vi "Write Page General Properties.vi"(8 "error in (no error)":errorcluster, 10 "General Page Properties":T1, 11 ".NET Refnum in":refnum<k24>) -> (0 "error out":errorcluster, 3 ".NET Refnum out":refnum<k24>)   [LabVIEW 2015, in "Configuration Tool.lvlib"]
uses:
  Configuration Tool.lvlib
  NationalInstruments.VeriStand.XMLReader
  Custom Device Type Defs/Page Properties.ctl
  XML Controls/Path Cluster.ctl
  XML Controls/help.ctl
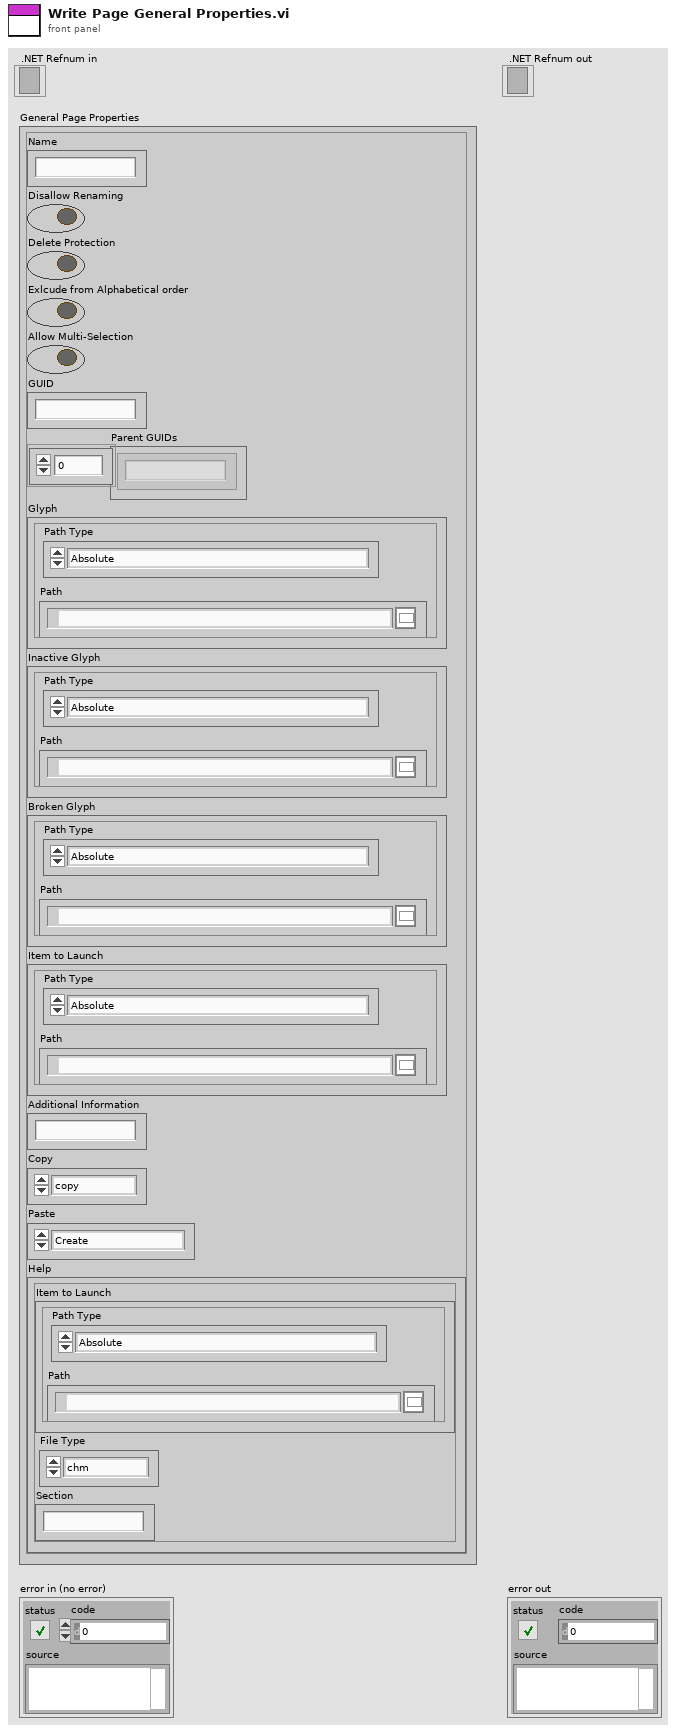
[diagram p1: front panel]
types:
  T1 = typedef "Page Properties.ctl" = cluster{"Name":string, "Disallow Renaming":bool, "Delete Protection":bool, "Exlcude from Alphabetical order":bool, "Allow Multi-Selection":bool, "GUID":string, "Parent GUIDs":string[], "Glyph":T2, "Inactive Glyph":T2, "Broken Glyph":T2, "Item to Launch":T2, "Additional Information":string, "Copy":enum16{"copy", "disabled"}, "Paste":enum16{"Create", "CreatIfNotExists_GUID", "CreatIfNotExists_Name", "Replace", "Dialog"}, "Help":T3}
  T2 = typedef "Configuration Tool.lvlib/Path Cluster.ctl" = cluster{"Path":path, "Path Type":enum16{"Absolute", "To Base", "To Common Doc Dir", "To Application Data Dir"}}
  T3 = typedef "Configuration Tool.lvlib/help.ctl" = cluster{"Item to Launch":T2, "Section":string, "File Type":enum16{"chm", "other"}}
  T4 = enum16{"Create", "CreatIfNotExists_GUID", "CreatIfNotExists_Name", "Replace", "Dialog"}
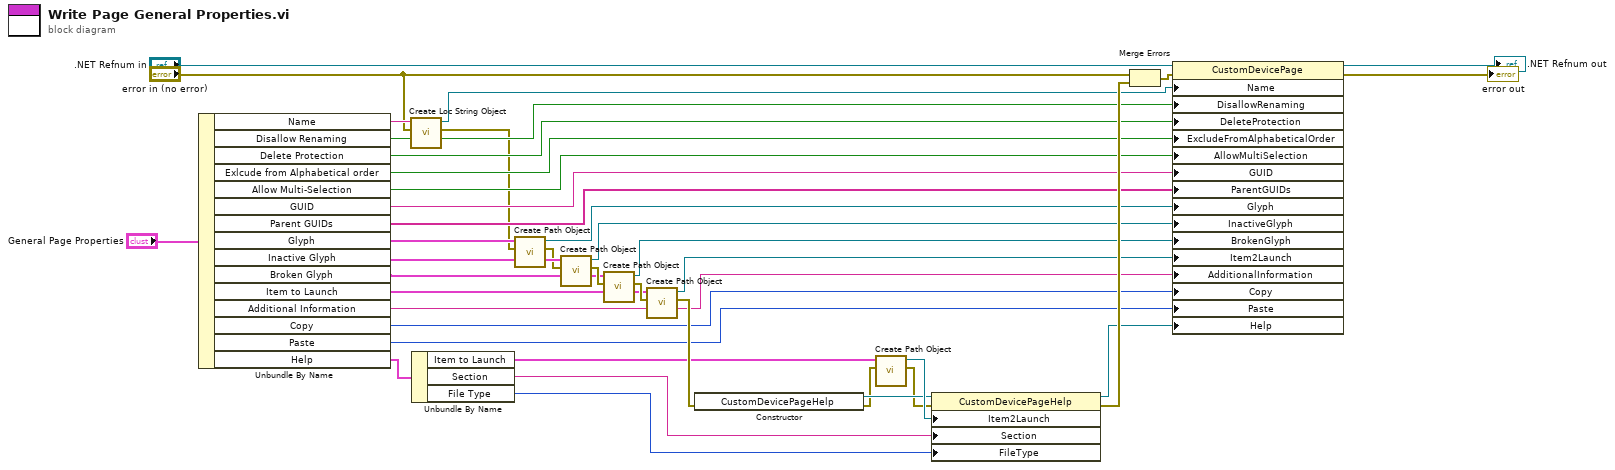
[diagram p0: block diagram]
diagram:
  n1 = Unbundle By Name("General Page Properties") -> ("Name"=w5:string, "Disallow Renaming"=w7:bool, "Delete Protection"=w8:bool, "Exlcude from Alphabetical order"=w9:bool, "Allow Multi-Selection"=w10:bool, "GUID"=w11:string, "Parent GUIDs"=w12:string[], "Glyph"=w13:T2, "Inactive Glyph"=w16:T2, "Broken Glyph"=w18:T2, "Item to Launch"=w21:T2, "Additional Information"=w24:string, "Copy"=w25:enum16{"copy", "disabled"}, "Paste"=w26:T4, "Help"=w27:T3)
  n2 = call "Create Loc String Object.vi"("error in (no error)"="error in (no error)", "Name"=w5) -> ("error out"=w1:errorcluster, ".NET Refnum out"=w6:refnum<k24>)  [unwired: 8 in]
  n3 = Unbundle By Name(w27) -> ("Item to Launch"=w28:T2, "Section"=w34:string, "File Type"=w35:enum16{"chm", "other"})
  n4 = call "Create Path Object.vi"("error in (no error)"=w1, "Path Info"=w13) -> ("error out"=w15:errorcluster, ".NET Refnum out"=w14:refnum<k24>)  [unwired: 8 in]
  n5 = call "Create Path Object.vi"("error in (no error)"=w15, "Path Info"=w16) -> ("error out"=w19:errorcluster, ".NET Refnum out"=w17:refnum<k24>)  [unwired: 8 in]
  n6 = call "Create Path Object.vi"("error in (no error)"=w19, "Path Info"=w18) -> ("error out"=w22:errorcluster, ".NET Refnum out"=w20:refnum<k24>)  [unwired: 8 in]
  n7 = call "Create Path Object.vi"("error in (no error)"=w22, "Path Info"=w21) -> ("error out"=w29:errorcluster, ".NET Refnum out"=w23:refnum<k24>)  [unwired: 8 in]
  n8 = constructor class="CustomDevicePageHelp"(error in=w29) -> (reference out=w32:refnum<k24>, error out=w30:errorcluster)  [unwired: 2 in, 1 out]
  n9 = call "Create Path Object.vi"("error in (no error)"=w30, "Path Info"=w28) -> ("error out"=w31:errorcluster, ".NET Refnum out"=w33:refnum<k24>)  [unwired: 8 in]
  n10 = property class="CustomDevicePageHelp"(reference=w32, error in=w31, "Item2Launch"=w33, "Section"=w34, "FileType"=w35) -> (reference out=w36:refnum<k24>, error out=w38:errorcluster)
  n11 = Merge Errors("error in (no error)", w38) -> (w37:errorcluster)
  n12 = property class="CustomDevicePage"(reference=".NET Refnum in", error in=w37, "Name"=w6, "DisallowRenaming"=w7, "DeleteProtection"=w8, "ExcludeFromAlphabeticalOrder"=w9, "AllowMultiSelection"=w10, "GUID"=w11, "ParentGUIDs"=w12, "Glyph"=w14, "InactiveGlyph"=w17, "BrokenGlyph"=w20, "Item2Launch"=w23, "AdditionalInformation"=w24, "Copy"=w25, "Paste"=w26, "Help"=w36) -> (reference out=→".NET Refnum out":refnum<k24>, error out=→"error out":errorcluster)
